vi "2 RIO.vi"   [LabVIEW 2011]
uses:
  2 Globals/2 Global.vi
types:
  T1 = typedef "UTM Location.ctl" = cluster{"UTM Zone":dbl, "Hemisphere":enum16{"North", "South"}, "East":dbl, "North":dbl}
  T2 = typedef "Velocity.ctl" = cluster{"East":dbl, "North":dbl}
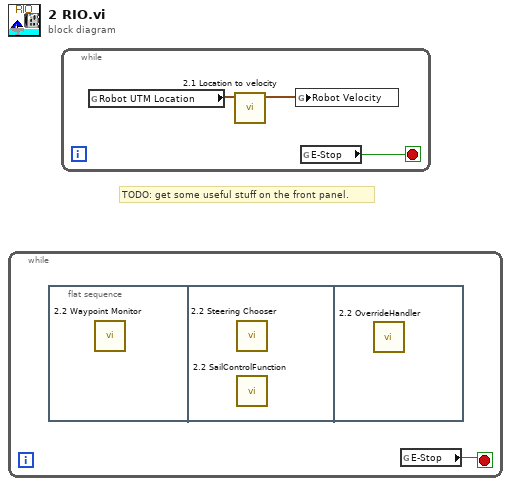
[diagram p0: block diagram]
diagram:
  # "TODO: get some useful stuff on the front panel."
  n1 = while {
    stop <- w1 stop-if-true
    n2 = flat-sequence {
      frame #0 {
        n3 = call "2.2 Waypoint Monitor.vi"() -> ()  [unwired: 12 in]
      }
      frame #1 {
        n4 = call "2.2 Steering Chooser.vi"() -> ()  [unwired: 12 in]
        n5 = call "2.2 SailControlFunction.vi"() -> ()  [unwired: 12 in]
      }
      frame #2 {
        n6 = call "2.2 OverrideHandler.vi"() -> ()  [unwired: 12 in]
      }
    }
    n7 = global read "2 Global.vi" "E-Stop"() -> (w1:bool)
  }
  n8 = while {
    stop <- w2 stop-if-true
    n9 = global read "2 Global.vi" "Robot UTM Location"() -> (w3:T1)
    n10 = call "2.1 Location to velocity.vi"("Robot UTM Location"=w3) -> ("Velocity"=w4:T2)  [unwired: 10 in]
    n11 = global write "2 Global.vi" "Robot Velocity"(w4) -> ()
    n12 = global read "2 Global.vi" "E-Stop"() -> (w2:bool)
  }
